vi "FastCMOS_EstimateOffsetGain.vi"() -> ()   [LabVIEW 2011]
uses:
  FastCMOS.llb/CameraConfig.ctl
  BeadTracker2.llb/GenericCameraConfigType.ctl
  <vilib>/Analysis/6fits.llb/Curve Fitting Criteria.ctl
  <vilib>/Analysis/NI_AALPro.lvlib
  <vilib>/vision/NI_Vision_Development_Module.lvlib
  <vilib>/Analysis/NI_AALBase.lvlib
panel:
  out "Waveform Chart":sgl(graph)
  out "Histogram Report":T1 {"Standard  Variation" format="%.2f"; "Mean Value" format="%.2f"; "Interval Width" format="%.2f"; "Starting Value" format="%.2f"; "Maximal Value" format="%.2f"; "Minimal Value" format="%.2f"}
  in  "Normal grab":bool
  out "gain mean":dbl format="%0.2f"
  out "gain min":dbl
  out "gain max":dbl
  out "Histogram":u32[](graph)
  out "Minimal Value":sgl
  out "Maximal Value":sgl
  in  "Base path":path
  in  "Image base name":string="camera_calib_"
  out "Buffer Number":i32
  out "Actual Width":u32
  out "Actual Height":u32
  out "Intercept":sgl[][](graph)
  out "Mean pixel val\nper intensity level":sgl[][][](array[numeric])
  in  "Stop":bool
  in  "Tab Control":T2(tab)
  out "Offsets":sgl[][](graph)
  in  "Number of darkframes":i32=300
  in  "Estimate offset/variance":bool
  out "Gain":sgl[][](graph)
  in  "Estimate gain":bool
  out "Wanted ET":i32
  out "Exposure level #":i32
  in  "# Exposure levels":i32=10
  in  "Max exposure time":i32=5000
  in  "Min exposure time":i32=50
  in  "Number of images\nper intensity level":i32=200
  out "Actual ET":i32
  out "Frame #":i32
  in  "Display image":bool
  out "Image":T3(plugin-control)
  in  "Camera settings (in)":T4={"Gain [1-4]"=1.0, "Offset"=128, "Mode"=6, "ROIs"=[{"X"=0, "Y"=0}], "ROI Size"={"X"=1280, "Y"=1024}, "Number of buffers"=40, "Use hardware multiple-ROI?"=FALSE, "GenericCameraConfig"={"Framerate (Hz)"=100, "Exposure time (us)"=3000, "Image size"={"Width"=1280, "Height"=1024}}} {"Mode" min=50}
  # "Run will also save to path\nentered above"
  # "Run will also save to path\nentered above"
  # "us"
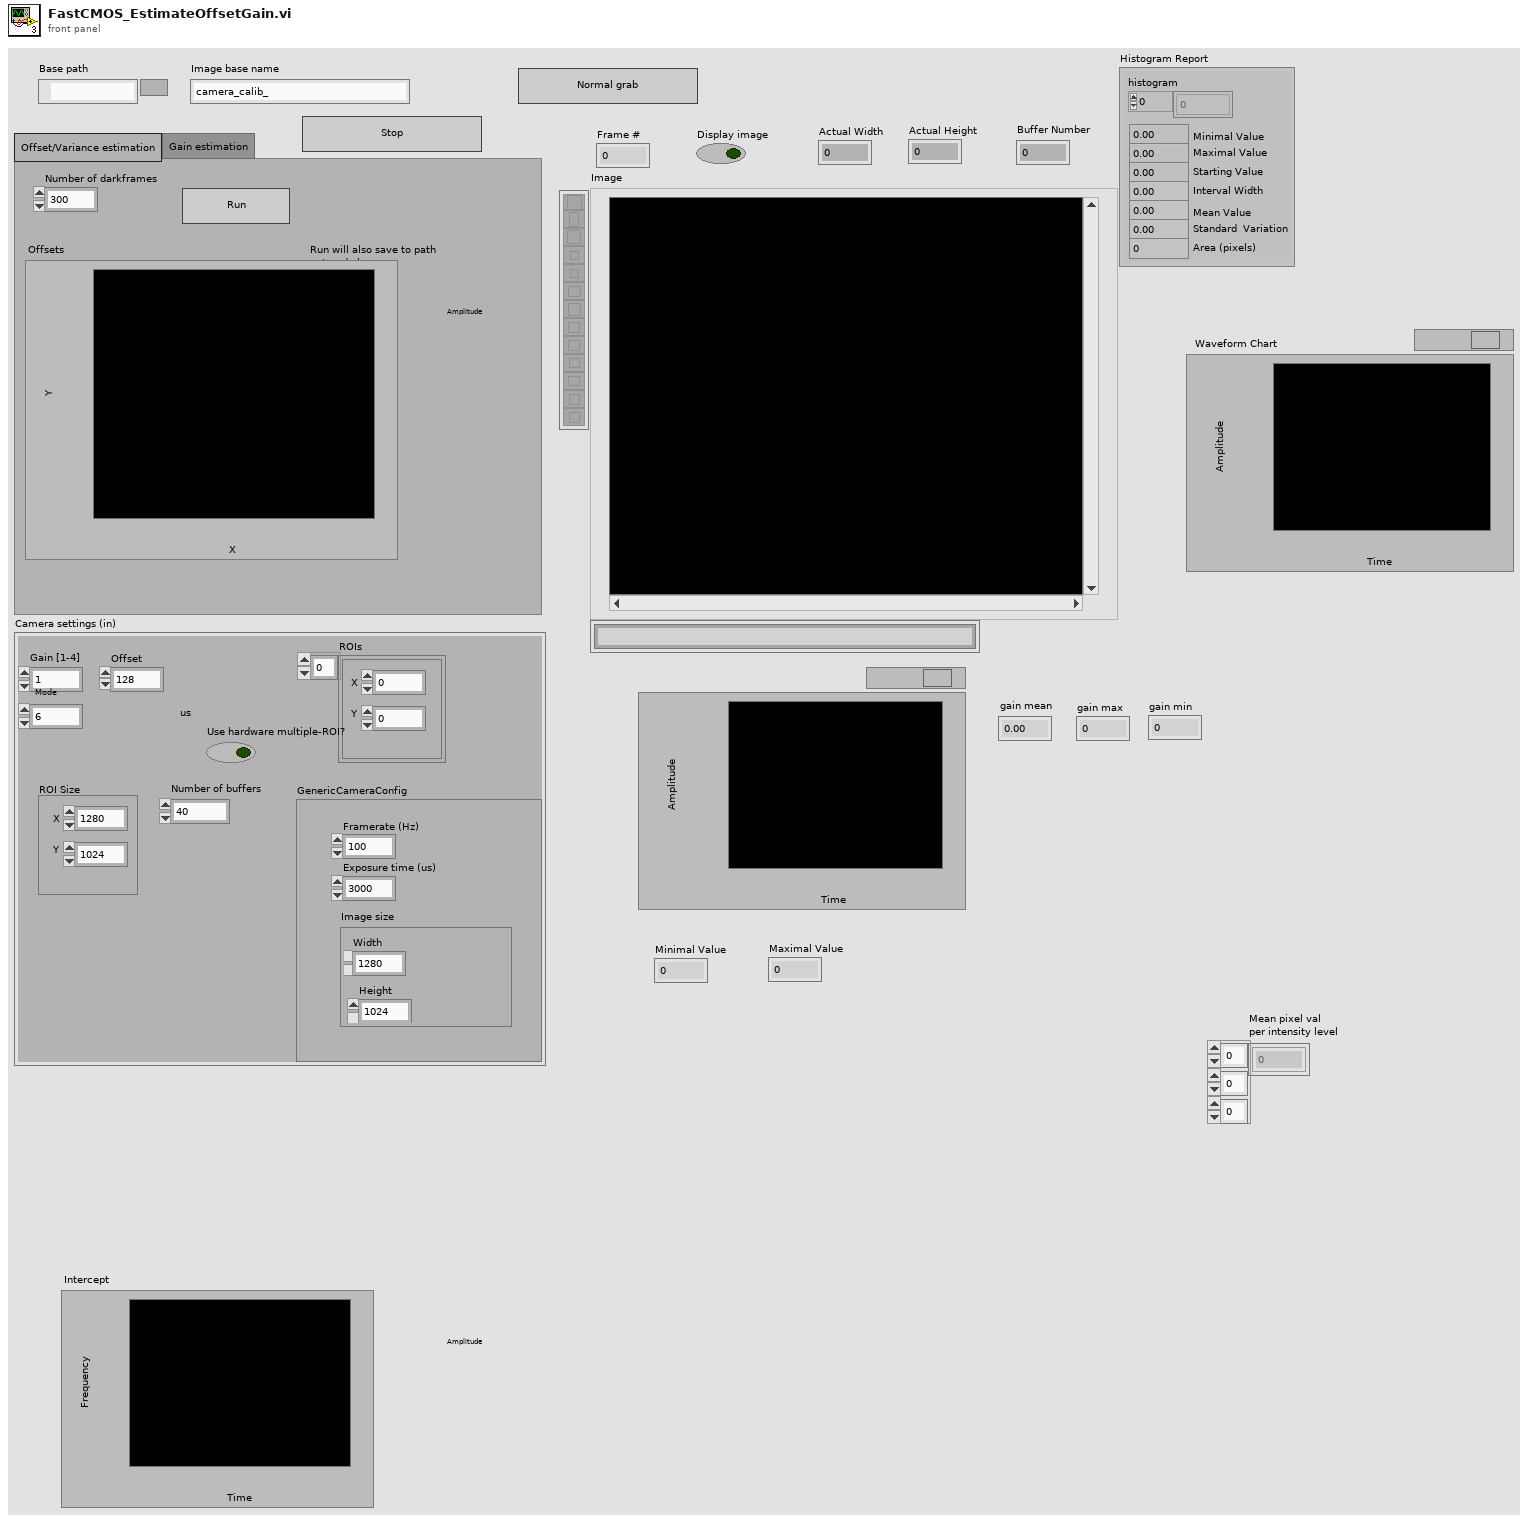
[diagram p1: front panel]
types:
  T1 = cluster{"histogram":u32[], "Minimal Value":sgl, "Maximal Value":sgl, "Starting Value":sgl, "Interval Width":sgl, "Mean Value":sgl, "Standard  Variation":sgl, "Area (pixels)":i32}
  T2 = enum32{"Offset/Variance estimation", "Gain estimation"}
  T3 = typedef "IMAQ Image.ctl" = refnum<image>
  T4 = typedef "CameraConfig.ctl" = cluster{"Gain [1-4]":sgl, "Offset":i16, "Mode":i16, "ROIs":cluster{"X":i32, "Y":i32}[], "ROI Size":cluster{"X":i32, "Y":i32}, "Number of buffers":i32, "Use hardware multiple-ROI?":bool, "GenericCameraConfig":T5}
  T5 = typedef "GenericCameraConfigType.ctl" = cluster{"Framerate (Hz)":i32, "Exposure time (us)":i32, "Image size":cluster{"Width":i32, "Height":i32}}
  T6 = enum16{"big-endian, network order", "native, host order", "little-endian"}
  T7 = enum16{"None", "Normalize", "NormalizeWithoutOffset"}
  T8 = typedef "NI_AALPro.lvlib/Curve Fitting Criteria.ctl" = u16
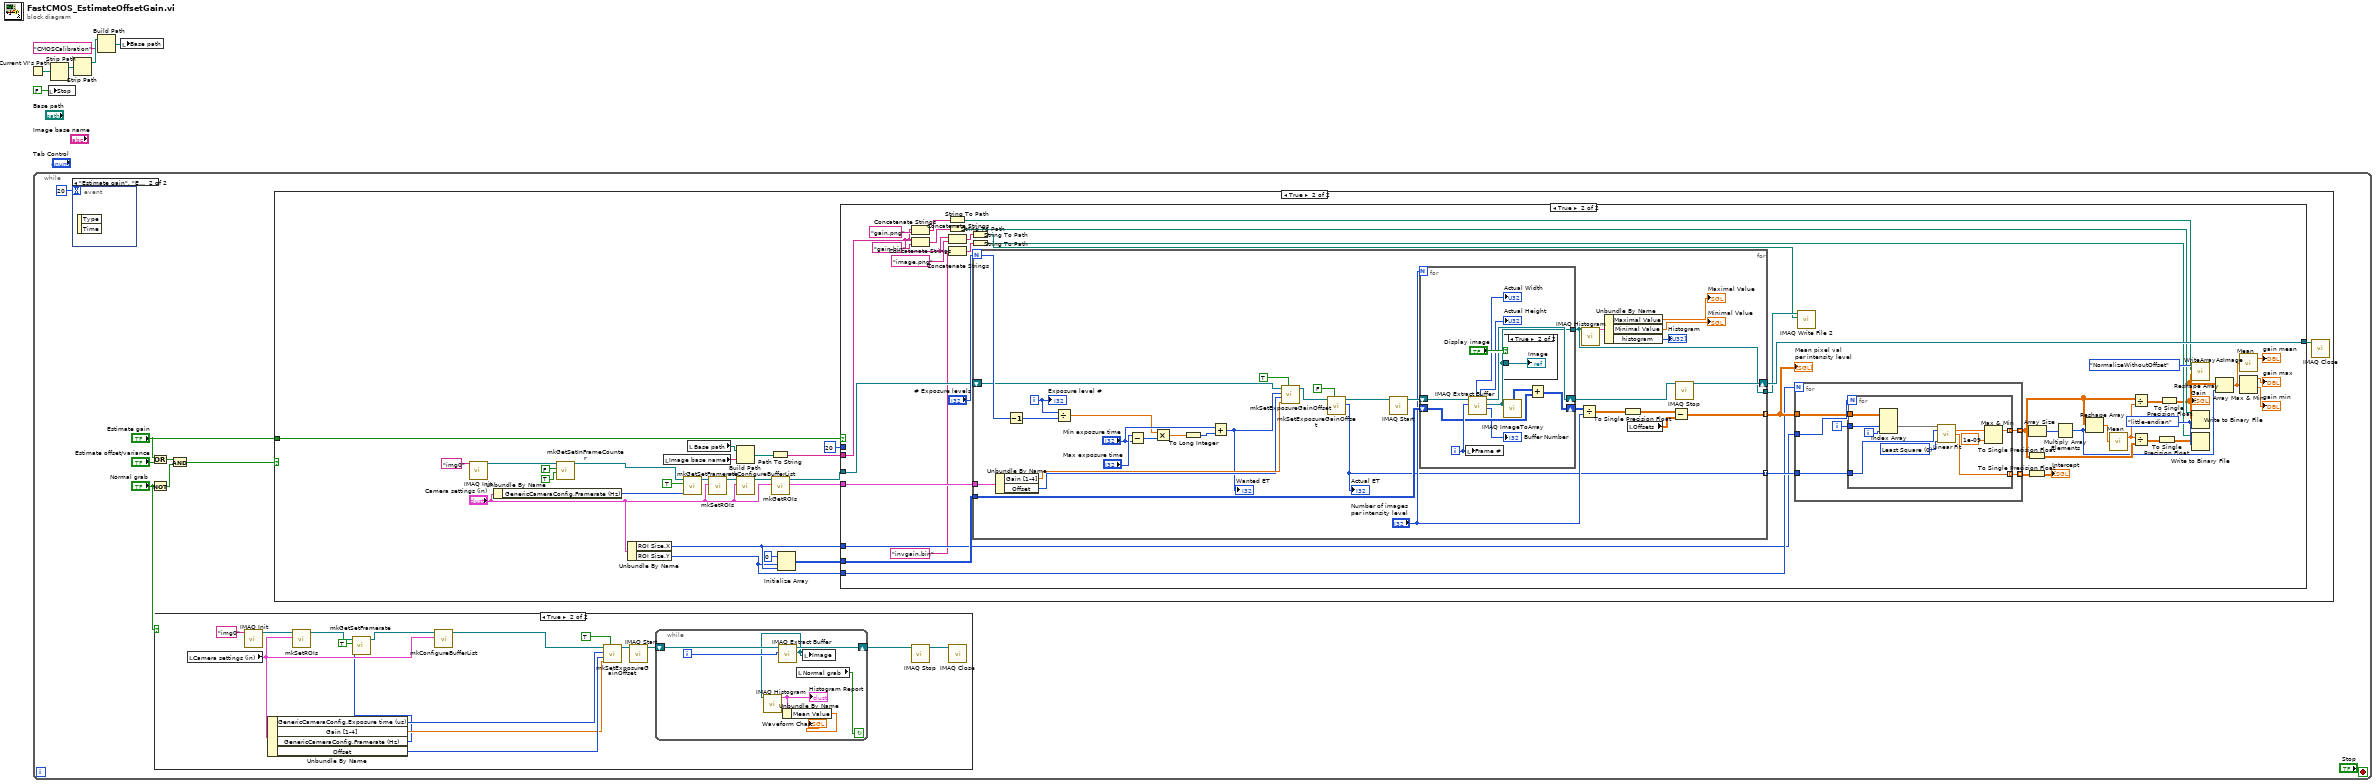
[diagram p0: block diagram]
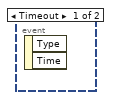
[diagram p3: hidden frame]
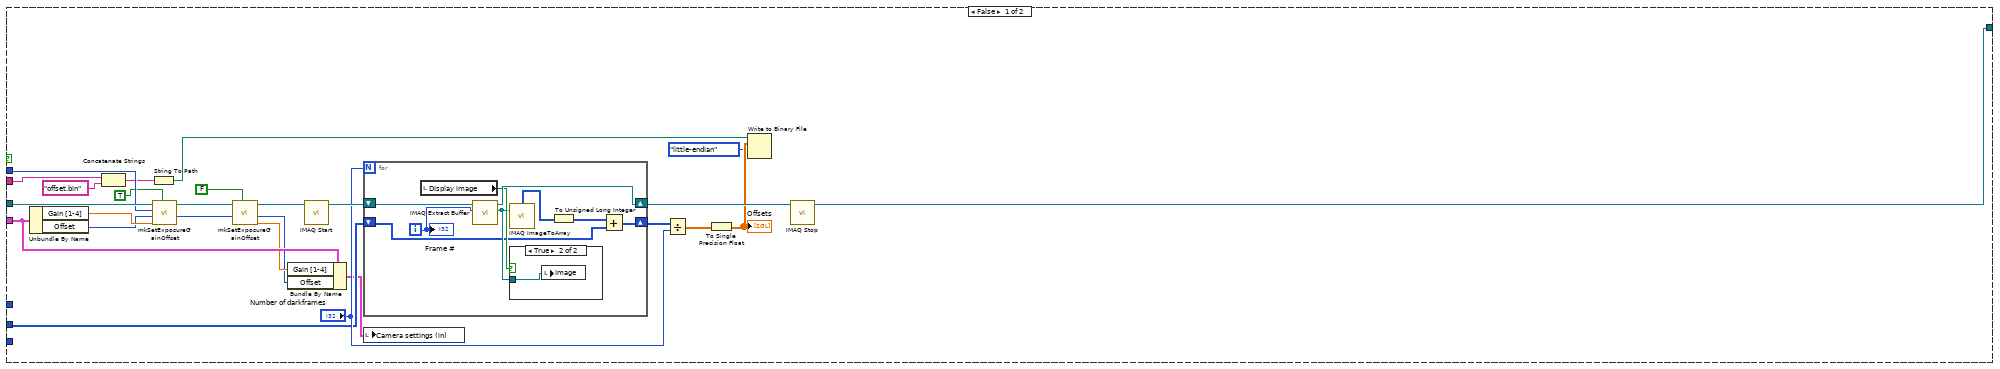
[diagram p5: hidden frame]
diagram:
  n1 = Current VI's Path() -> (path=w5:path)
  n2 = while {
    stop <- "Stop" stop-if-true
    n3 = event shown="[1] \"Estimate gain\", \"Estimate offset/variance\": Value Change" {
      selector: _ -> [_ _]
      dyn-events: _ -> [_ _]
      timeout: 20 -> [_ _]
      event Timeout {
        n4 = event-data() -> ()  [unwired: 1 in, 2 out]
      }
      event "Estimate gain", "Estimate offset/variance": Value Change {
        n5 = event-data() -> ()  [unwired: 1 in, 2 out]
      }
    }
    n6 = Or(x="Estimate gain", y="Estimate offset/variance") -> (x .or. y?=w10:bool)
    n7 = Not(x="Normal grab") -> (.not. x?=w9:bool)
    n8 = case shown="True" "Normal grab" {
      frame False {
      }
      frame True {
        n9 = local read "Camera settings (in)"() -> (w24:T4)
        n10 = call <vilib>:"IMAQ Init.vi"("Interface Name"="img0") -> ("IMAQ Session Out"=w26:refnum<k11>)  [unwired: 9 in, 1 out]
        n11 = Unbundle By Name(w24) -> ("GenericCameraConfig.Exposure time (us)"=w23:i32, "Gain [1-4]"=w20:sgl, "GenericCameraConfig.Framerate (Hz)"=w15:i32, "Offset"=w22:i16)
        n12 = call "mkSetROIs.vi"("Camera in"=w24, "IMAQ Refnum in"=w26) -> ("IMAQ Refnum out"=w18:refnum<k11>)  [unwired: 9 in]
        n13 = call "mkGetSetFramerate.vi"("Framerate"=w15, "Set? (F)"=TRUE, "IMAQ Refnum out"=w18) -> ("IMAQ Refnum (out)"=w17:refnum<k11>)  [unwired: 5 in, 3 out]
        n14 = call "mkConfigureBufferList.vi"("Camera in"=w24, "IMAQ Session"=w17) -> ("IMAQ Session (out)"=w25:refnum<k11>)  [unwired: 9 in]
        n15 = call "mkSetExposureGainOffset.vi"("Set? (F)"=TRUE, "Gain [1-4]"=w20, "Offset"=w22, "Exposure time"=w23, "IMAQ Refnum in"=w25) -> ("IMAQ Refnum out"=w21:refnum<k11>)  [unwired: 1 in, 5 out]
        n16 = call <vilib>:"IMAQ Start.vi"("IMAQ Session In"=w21) -> ("IMAQ Session Out"=w29:refnum<k11>)  [unwired: 9 in, 1 out]
        n17 = while {
          shift-right: [w34] -> w28
          shift-left: w29 -> [w35]
          i -> [w36]
          stop <- w37 continue-if-true
          n18 = call <vilib>:"IMAQ Extract Buffer.vi"("Buffer to extract"=w36, "IMAQ Session In"=w35) -> ("Image Out"=w33:T3, "IMAQ Session Out"=w34:refnum<k11>)  [unwired: 4 in, 4 out]
          n19 = call "IMAQ Histogram"("Image"=w33) -> ("Histogram Report"=w32:T1)  [unwired: 9 in, 1 out]
          "Histogram Report" <- w32
          n20 = Unbundle By Name(w32) -> ("Mean Value"=→"Waveform Chart":sgl)
          n21 = local read "Normal grab"() -> (w37:bool)
          n22 = local write "Image"(w33) -> ()
        }
        n23 = call <vilib>:"IMAQ Stop.vi"("IMAQ Session In"=w28) -> ("IMAQ Session Out"=w27:refnum<k11>)  [unwired: 9 in, 1 out]
        n24 = call <vilib>:"IMAQ Close.vi"("IMAQ Session In"=w27) -> ()  [unwired: 10 in, 1 out]
      }
    }
    n25 = And(x=w10, y=w9) -> (x .and. y?=w8:bool)
    n26 = case shown="True" w8 {
      tunnel: "Estimate gain" -> [_ w51]
      frame False {
      }
      frame True {
        n27 = call <vilib>:"IMAQ Init.vi"("Interface Name"="img0") -> ("IMAQ Session Out"=w56:refnum<k11>)  [unwired: 9 in, 1 out]
        n28 = Unbundle By Name("Camera settings (in)") -> ("GenericCameraConfig.Framerate (Hz)"=w52:i32)
        n29 = call "mkGetSetInFrameCounter.vi"("Set? (F)"=TRUE, "Enable in-frame counter (T)"=FALSE, "IMAQ Refnum in"=w56) -> ("IMAQ Refnum out"=w55:refnum<k11>)  [unwired: 7 in, 1 out]
        n30 = Unbundle By Name("Camera settings (in)") -> ("ROI Size.X"=w48:i32, "ROI Size.Y"=w47:i32)
        n31 = local read "Image base name"() -> (w42:string)
        n32 = call "mkGetSetFramerate.vi"("Framerate"=w52, "Set? (F)"=TRUE, "IMAQ Refnum out"=w55) -> ("IMAQ Refnum (out)"=w60:refnum<k11>)  [unwired: 5 in, 3 out]
        n33 = local read "Base path"() -> (w43:path)
        n34 = call "mkSetROIs.vi"("Camera in"="Camera settings (in)", "IMAQ Refnum in"=w60) -> ("IMAQ Refnum out"=w59:refnum<k11>)  [unwired: 9 in]
        n35 = Build Path(base path=w43, name or relative path=w42) -> (appended path=w41:path)
        n36 = call "mkConfigureBufferList.vi"("Camera in"="Camera settings (in)", "IMAQ Session"=w59) -> ("IMAQ Session (out)"=w46:refnum<k11>)  [unwired: 9 in]
        n37 = Path To String(path=w41) -> (string=w40:string)
        n38 = call "mkGetROIs.vi"("Camera settings"="Camera settings (in)", "IMAQ Refnum in"=w46) -> ("Camera settings (out)"=w44:T4, "IMAQ Refnum out"=w45:refnum<k11>)  [unwired: 8 in]
        n39 = Initialize Array(u32 0 ("element"), w47, w48) -> (w49:u32[][])
        n40 = case shown="True" w51 {
          tunnel: w45 -> [w87 w137]
          tunnel: [w84 w136] -> w58
          tunnel: w44 -> [w71 w134]
          tunnel: w49 -> [w80 w135]
          tunnel: w48 -> [_ w130]
          tunnel: w47 -> [_ w131]
          tunnel: 20 ("GenericCameraConfig.Exposure time (us)") -> [w76 _]
          tunnel: w40 -> [w66 w106]
          frame False {
            n41 = Unbundle By Name(w71) -> ("Gain [1-4]"=w75:sgl, "Offset"=w74:i16)
            n42 = Concatenate Strings(w66, "offset.bin" ("string")) -> (w65:string)
            n43 = String To Path(string=w65) -> (path=w64:path)
            n44 = call "mkSetExposureGainOffset.vi"("Set? (F)"=TRUE, "Gain [1-4]"=w75, "Offset"=w74, "Exposure time"=w76, "IMAQ Refnum in"=w87) -> ("Offset"=w77:u32, "IMAQ Refnum out"=w79:refnum<k11>)  [unwired: 1 in, 4 out]
            n45 = call "mkSetExposureGainOffset.vi"("Set? (F)"=FALSE, "Offset"=w77, "IMAQ Refnum in"=w79) -> ("Gain"=w70:dbl, "Offset"=w69:u32, "IMAQ Refnum out"=w78:refnum<k11>)  [unwired: 3 in, 3 out]
            n46 = Bundle By Name(cluster=w71, "Gain [1-4]"=w70, "Offset"=w69) -> (w68:T4)
            n47 = call <vilib>:"IMAQ Start.vi"("IMAQ Session In"=w78) -> ("IMAQ Session Out"=w86:refnum<k11>)  [unwired: 9 in, 1 out]
            n48 = for {
              N: "Number of darkframes" -> [_]
              shift-right: [w94] -> w85
              shift-left: w86 -> [w96]
              shift-right: [w88] -> w83
              shift-left: w80 -> [w89]
              i -> [w95]
              n49 = local read "Display image"() -> (w93:bool)
              n50 = call <vilib>:"IMAQ Extract Buffer.vi"("Buffer to extract"=w95, "IMAQ Session In"=w96) -> ("Image Out"=w92:T3, "IMAQ Session Out"=w94:refnum<k11>)  [unwired: 4 in, 4 out]
              n51 = call "IMAQ ImageToArray"("Image"=w92) -> ("Image Pixels (U8)"=w91:u8[][])  [unwired: 3 in, 4 out]
              n52 = case shown="True" w93 {
                tunnel: w92 -> [_ w97]
                frame False {
                }
                frame True {
                  n53 = local write "Image"(w97) -> ()
                }
              }
              n54 = To Unsigned Long Integer(number=w91) -> (unsigned 32bit integer=w90:u32[][])
              n55 = Add(x=w90, y=w89) -> (x+y=w88:u32[][])
              "Frame #" <- w95
            }
            n56 = local write "Camera settings (in)"(w68) -> ()
            n57 = Divide(x=w83, y="Number of darkframes") -> (x/y=w81:dbl[][])
            n58 = To Single Precision Float(number=w81) -> (single precision float=w63:sgl[][])
            "Offsets" <- w63
            n59 = Write to Binary File(file (use dialog)=w64, data=w63, 9:T6."little-endian" ("byte order (0:big-endian, network order)")) -> ()  [unwired: 3 in, 3 out]
            n60 = call <vilib>:"IMAQ Stop.vi"("IMAQ Session In"=w85) -> ("IMAQ Session Out"=w84:refnum<k11>)  [unwired: 9 in, 1 out]
          }
          frame True {
            w104 = T6."little-endian" ("byte order (0:big-endian, network order)")
            n61 = Concatenate Strings(w106, "gain.png" ("string")) -> (w118:string)
            n62 = Concatenate Strings(w106, "gain.bin" ("string")) -> (w120:string)
            n63 = String To Path(string=w118) -> (path=w117:path)
            n64 = String To Path(string=w120) -> (path=w119:path)
            n65 = Concatenate Strings(w106, "image.png" ("string")) -> (w123:string)
            n66 = Concatenate Strings(w106, "invgain.bin" ("string")) -> (w105:string)
            n67 = String To Path(string=w123) -> (path=w122:path)
            n68 = String To Path(string=w105) -> (path=w103:path)
            n69 = for {
              N: "# Exposure levels" -> [w185]
              tunnel: w134 -> [w166]
              shift-right: [w176] -> w136
              shift-left: w137 -> [w179]
              tunnel: w135 -> [w175]
              tunnel: [w169] -> w133 mode=indexing
              tunnel: [w163] -> w132 mode=indexing
              tunnel: [w155] -> w125
              i -> [w186]
              n70 = Unbundle By Name(w166) -> ("Gain [1-4]"=w165:sgl, "Offset"=w164:i16)
              n71 = Decrement(x=w185) -> (x-1=w184:i32)
              n72 = Divide(x=w186, y=w184) -> (x/y=w183:dbl)
              n73 = Subtract(x="Max exposure time", y="Min exposure time") -> (x-y=w182:i32)
              n74 = Multiply(x=w183, y=w182) -> (x*y=w181:dbl)
              n75 = To Long Integer(number=w181) -> (32bit integer=w180:i32)
              n76 = Add(x="Min exposure time", y=w180) -> (x+y=w162:i32)
              "Wanted ET" <- w162
              n77 = call "mkSetExposureGainOffset.vi"("Set? (F)"=TRUE, "Gain [1-4]"=w165, "Offset"=w164, "Exposure time"=w162, "IMAQ Refnum in"=w179) -> ("IMAQ Refnum out"=w168:refnum<k11>)  [unwired: 1 in, 5 out]
              n78 = call "mkSetExposureGainOffset.vi"("Set? (F)"=FALSE, "IMAQ Refnum in"=w168) -> ("Exposure time"=w163:i32, "IMAQ Refnum out"=w167:refnum<k11>)  [unwired: 4 in, 4 out]
              "Actual ET" <- w163
              n79 = call <vilib>:"IMAQ Start.vi"("IMAQ Session In"=w167) -> ("IMAQ Session Out"=w178:refnum<k11>)  [unwired: 9 in, 1 out]
              n80 = for {
                N: "Number of images\nper intensity level" -> [_]
                shift-right: [w197] -> w177
                shift-left: w178 -> [w198]
                shift-right: [w193] -> w174
                shift-left: w175 -> [w194]
                tunnel: [w189] -> w155
                i -> [w196]
                n81 = local write "Frame #"(w196) -> ()
                n82 = call <vilib>:"IMAQ Extract Buffer.vi"("Buffer to extract"=w196, "IMAQ Session In"=w198) -> ("Buffer Number"=→"Buffer Number":i32, "Image Out"=w189:T3, "IMAQ Session Out"=w197:refnum<k11>, "Actual Height"=→"Actual Height":u32, "Actual Width"=→"Actual Width":u32)  [unwired: 4 in, 1 out]
                n83 = case shown="True" "Display image" {
                  tunnel: w189 -> [_ w200]
                  frame False {
                  }
                  frame True {
                    "Image" <- w200
                  }
                }
                n84 = call "IMAQ ImageToArray"("Image"=w189) -> ("Image Pixels (U8)"=w195:u8[][])  [unwired: 3 in, 4 out]
                n85 = Add(x=w195, y=w194) -> (x+y=w193:u32[][])
              }
              n86 = Divide(x=w174, y="Number of images\nper intensity level") -> (x/y=w172:dbl[][])
              n87 = call "IMAQ Histogram"("Image"=w155) -> ("Histogram Report"=w159:T1)  [unwired: 9 in, 1 out]
              n88 = Unbundle By Name(w159) -> ("Maximal Value"=→"Maximal Value":sgl, "Minimal Value"=→"Minimal Value":sgl, "histogram"=→"Histogram":u32[])
              n89 = To Single Precision Float(number=w172) -> (single precision float=w171:sgl[][])
              n90 = local read "Offsets"() -> (w170:sgl[][])
              n91 = Subtract(x=w171, y=w170) -> (x-y=w169:sgl[][])
              n92 = call <vilib>:"IMAQ Stop.vi"("IMAQ Session In"=w177) -> ("IMAQ Session Out"=w176:refnum<k11>)  [unwired: 9 in, 1 out]
              "Exposure level #" <- w186
            }
            "Mean pixel val\nper intensity level" <- w133
            n93 = for {
              N: w131 -> [_]
              tunnel: w130 -> [w144]
              tunnel: w133 -> [w143]
              tunnel: w132 -> [w141]
              tunnel: [w140] -> w101 mode=indexing
              tunnel: [w139] -> w129 mode=indexing
              i -> [w142]
              n94 = for {
                N: w144 -> [_]
                tunnel: w143 -> [w154]
                tunnel: w142 -> [w153]
                tunnel: w141 -> [w151]
                tunnel: [w145] -> w140 mode=indexing
                tunnel: [w148] -> w139 mode=indexing
                i -> [w152]
                w149 = T8 0 items=["Least Square", "Least Absolute Residual", "Bisquare"] ("method")
                n95 = Index Array(array=w154, index (dim 1)=w153, index (dim 2)=w152) -> (element=w150:sgl[])  [unwired: 1 in]
                n96 = call <vilib>:"Linear Fit.vi"("Y"=w150, "X"=w151, "method"=w149) -> ("slope"=w146:dbl, "intercept"=w148:dbl)  [unwired: 8 in, 3 out]
                n97 = Max & Min(x=w146, y=1e-09) -> (max(x,y)=w145:dbl)  [unwired: 1 out]
              }
            }
            n98 = call-poly "IMAQ Write File 2"("File Path"=w122, "Image"=w125) -> ()  [unwired: 8 in, 2 out]
            n99 = Array Size(array=w101) -> (size(s)=w116:i32[])
            n100 = To Single Precision Float(number=w101) -> (single precision float=w112:sgl[][])
            n101 = To Single Precision Float(number=w129) -> (single precision float=→"Intercept":sgl[][])
            n102 = Multiply Array Elements(1:w116) -> (0:w111:i32)
            n103 = Reshape Array(w101, w111) -> (w113:dbl[])
            n104 = call <vilib>:"Mean.vi"("X"=w113) -> ("mean"=w100:dbl)  [unwired: 1 out]
            n105 = Divide(x=w101, y=w100) -> (x/y=w99:dbl[][])
            n106 = Divide(x=w100, y=w112) -> (x/y=w108:dbl[][])
            n107 = To Single Precision Float(number=w108) -> (single precision float=w102:sgl[][])
            n108 = To Single Precision Float(number=w99) -> (single precision float=w98:sgl[][])
            "Gain" <- w98
            n109 = call "WriteArrayAsImage.vi"("Data"=w98, "File Path"=w117, "Normalize Mode"=T7."NormalizeWithoutOffset") -> ()  [unwired: 9 in]
            n110 = Write to Binary File(file (use dialog)=w119, data=w98, 9:w104) -> ()  [unwired: 3 in, 3 out]
            n111 = Write to Binary File(file (use dialog)=w103, data=w102, 9:w104) -> ()  [unwired: 3 in, 3 out]
            n112 = Reshape Array(w98, w111) -> (w110:sgl[])
            n113 = call <vilib>:"Mean.vi"("X"=w110) -> ("mean"=→"gain mean":dbl)  [unwired: 1 out]
            n114 = Array Max & Min(array=w110) -> (max value=→"gain max":sgl, min value=→"gain min":sgl)  [unwired: 2 out]
          }
        }
        n115 = call <vilib>:"IMAQ Close.vi"("IMAQ Session In"=w58) -> ()  [unwired: 10 in, 1 out]
      }
    }
  }
  n116 = local write "Stop"(FALSE ("Stop")) -> ()
  n117 = Strip Path(path=w5) -> (stripped path=w4:path)  [unwired: 1 out]
  n118 = Strip Path(path=w4) -> (stripped path=w3:path)  [unwired: 1 out]
  n119 = Build Path(base path=w3, name or relative path="CMOSCalibration") -> (appended path=w1:path)
  n120 = local write "Base path"(w1) -> ()
